vi "Get Dev Info.vi"() -> ()   [LabVIEW 2011]
uses:
  Private/DMGR/DMGR.lvlib
panel:
  out "DTP":u32
  out "Connection String":string
  out "Name":string
  out "Error Out":errorcluster
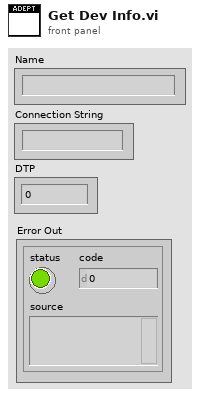
[diagram p1: front panel]
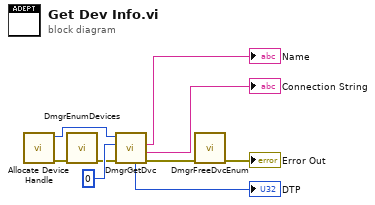
[diagram p0: block diagram]
diagram:
  n1 = call "Allocate Device Handle.vi"() -> ("Error Out"=w7:errorcluster, "Device Handle"=w9:u64)  [unwired: 10 in]
  n2 = call "DmgrEnumDevices.vi"("Error In"=w7) -> ("Error Out"=w6:errorcluster)  [unwired: 9 in, 1 out]
  n3 = call "DmgrGetDvc.vi"("Error In"=w6, "Device Number"=0, "Device Handle"=w9) -> ("Error Out"=w4:errorcluster, "Connection String"=→"Connection String":string, "Name"=→"Name":string, "DTP"=→"DTP":u32)  [unwired: 4 in, 1 out]
  n4 = call "DmgrFreeDvcEnum.vi"("Error In"=w4) -> ("Error Out"=→"Error Out":errorcluster)  [unwired: 10 in]
